vi "tcp 쓰기2.vi"() -> ()   [LabVIEW 2014]
panel:
  out "A":i16[](array[numeric])
  out "에러 출력":errorcluster
  out "문자 2":i16=-19239
  out "문자열":i16[](array[numeric])
  in  "불리언":bool
  out "참 거짓":string
  out "숫자":u32
  in  "stop":bool
  out "문자열":string
  out "Dato Leido":bool[](array[boolean])
  in  "stop 2":bool
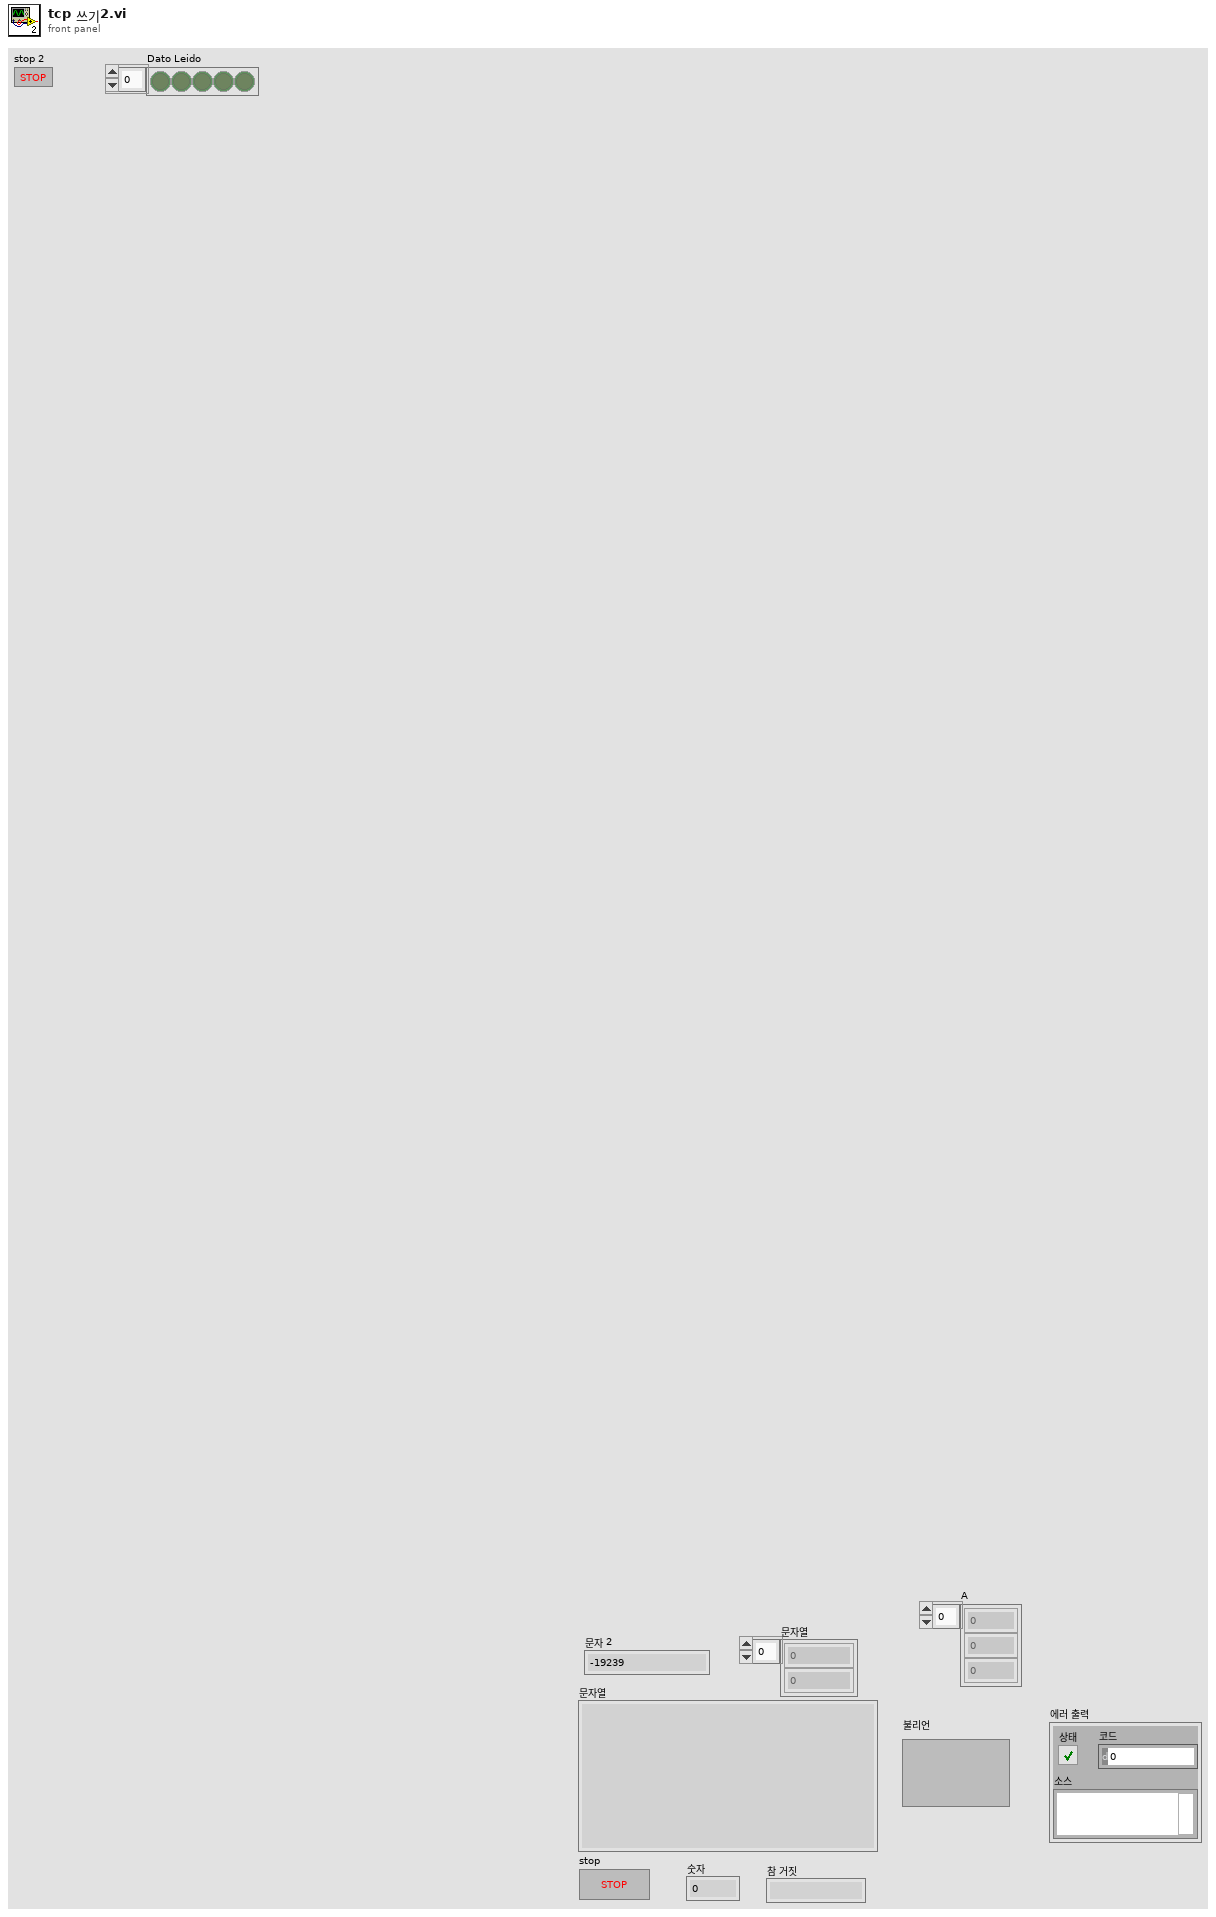
[diagram p1: front panel]
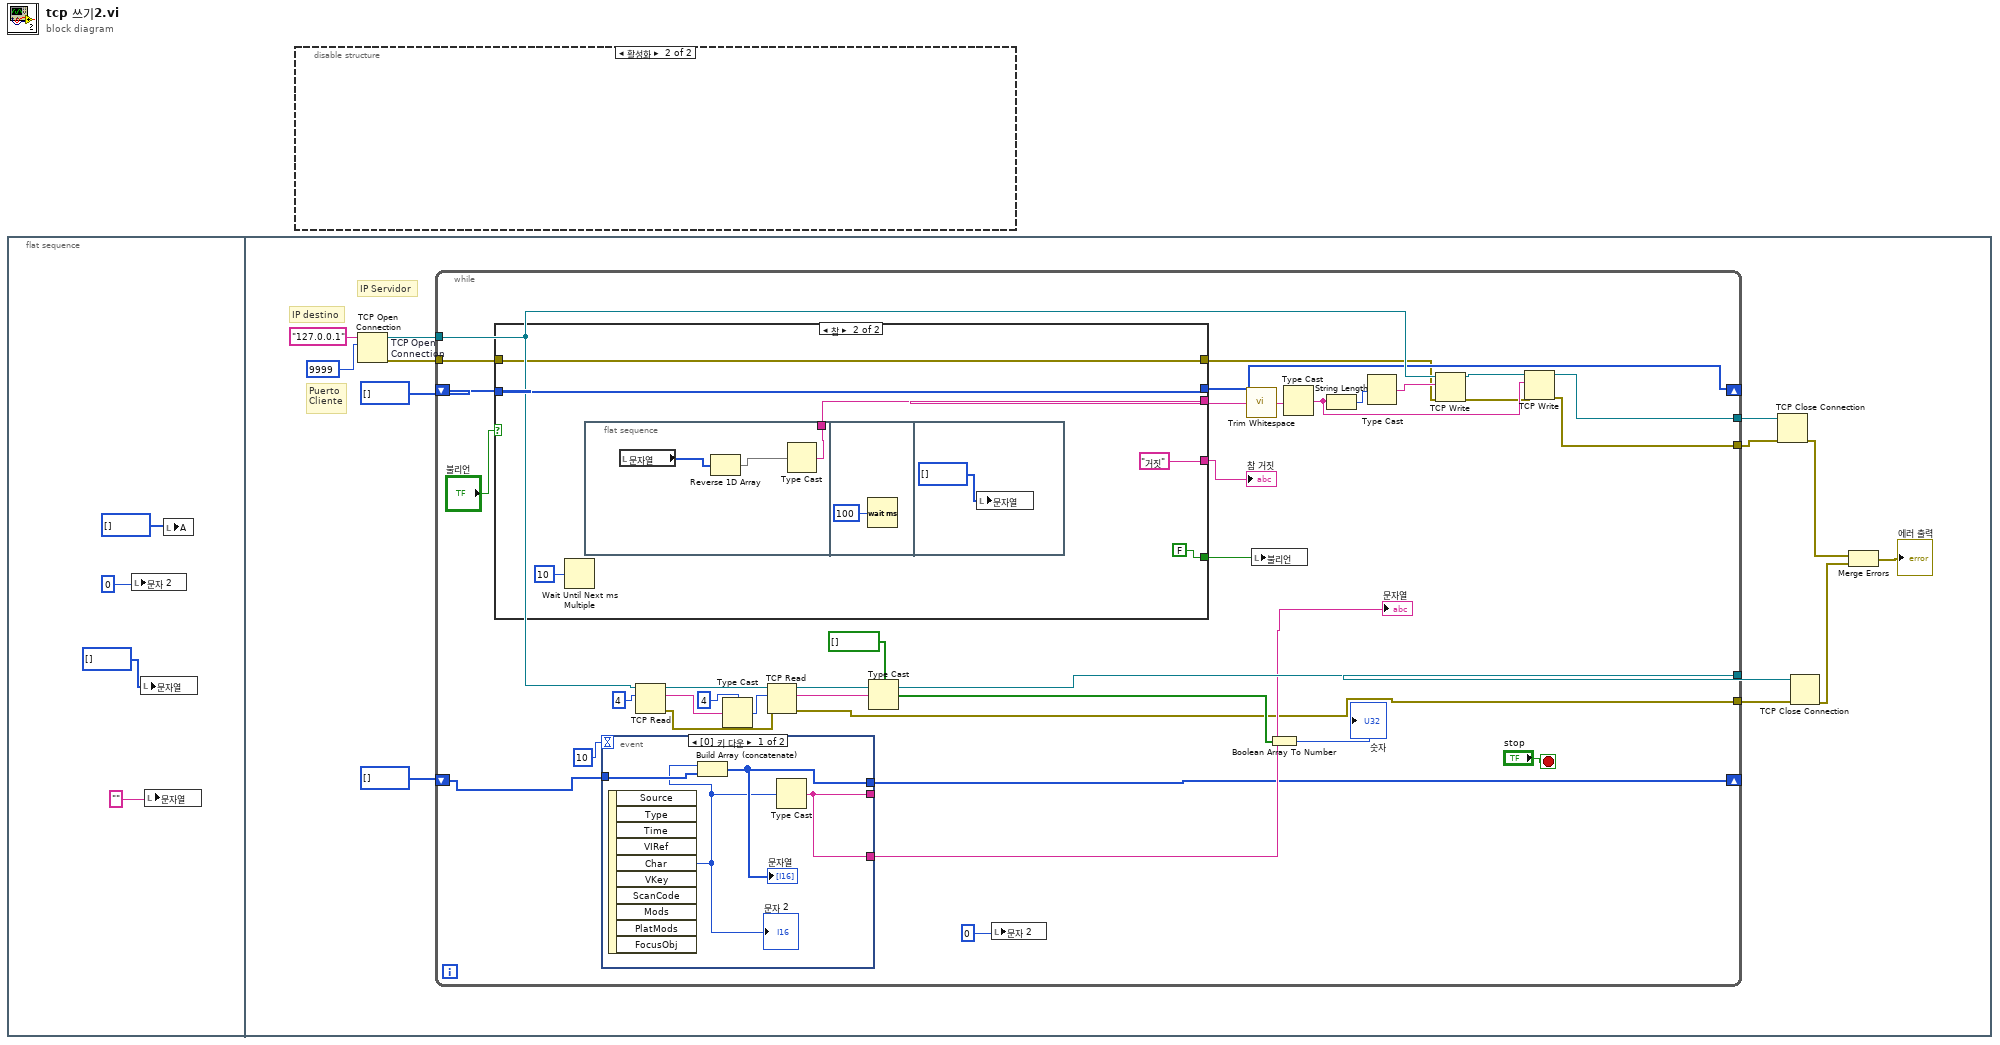
[diagram p0: block diagram]
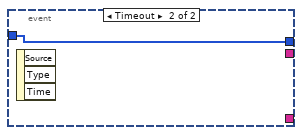
[diagram p2: hidden frame]
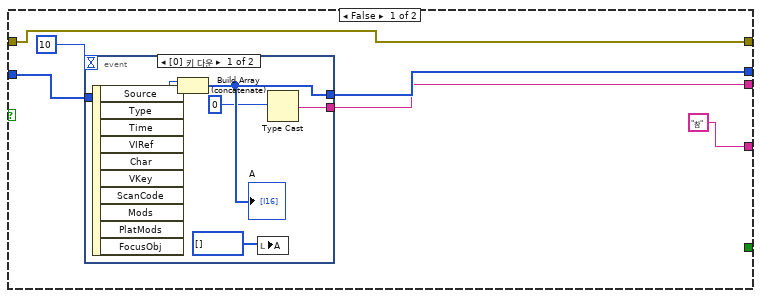
[diagram p3: hidden frame]
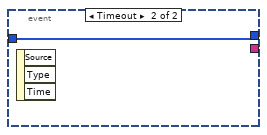
[diagram p4: hidden frame]
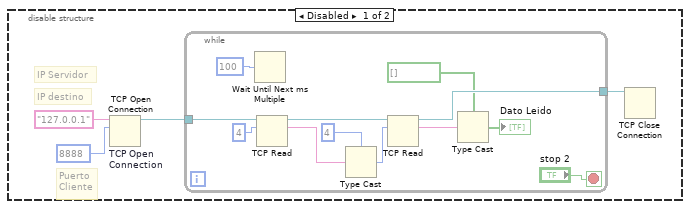
[diagram p5: hidden frame]
diagram:
  n1 = flat-sequence {
    frame #0 {
      n2 = local write "문자 2"(0) -> ()
      n3 = local write "문자열"(i16[] []) -> ()
      n4 = local write "문자열"("") -> ()
      n5 = local write "A"(i16[] []) -> ()
    }
    frame #1 {
      # "Puerto\nCliente"
      # "IP Servidor"
      # "IP destino"
      n6 = TCP Open Connection "TCP Open \nConnection"(address="127.0.0.1", remote port or service name=u16 9999) -> (connection ID=w17:refnum<k5>, error out=w10:errorcluster)  [unwired: 3 in]
      n7 = while {
        tunnel: w17 -> [w44]
        tunnel: [w52] -> w14
        shift-right: [w28] -> _
        shift-left: i16[] [] -> [w51]
        tunnel: [w41] -> w13
        shift-right: [w29] -> _
        shift-left: i16[] [] -> [w30]
        tunnel: w10 -> [w27]
        tunnel: [w24] -> w5
        tunnel: [w22] -> w8
        stop <- "stop" stop-if-true
        n8 = case shown="참" "불리언" {
          tunnel: w51 -> [w63 w76]
          tunnel: [w62 w76] -> w28
          tunnel: [_ FALSE ("불리언")] -> w33
          tunnel: [w60 w72] -> w20
          tunnel: w27 -> [w59 w73]
          tunnel: [w59 w73] -> w26
          tunnel: ["참" "거짓"] -> w18
          frame False {
            n9 = event shown="[0] 키 다운" {
              selector: _ -> [_ _]
              dyn-events: _ -> [_ _]
              timeout: 10 -> [_ _]
              tunnel: [w68 w70] -> w62
              tunnel: w63 -> [w69 w70]
              tunnel: [w66 _] -> w60
              event Key Down {
                n10 = event-data() -> ("Char"=w67:i16)  [unwired: 1 in, 9 out]
                n11 = Build Array (concatenate)(w67, w69) -> (w68:i16[])
                "A" <- w68
                n12 = local write "A"(i16[] []) -> ()
                n13 = Type Cast(x=0) -> (*(type *) &x=w66:string)  [unwired: 1 in]
              }
              event Timeout {
                n14 = event-data() -> ()  [unwired: 1 in, 3 out]
              }
            }
          }
          frame True {
            n15 = Wait Until Next ms Multiple(millisecond multiple=u32 10) -> ()  [unwired: 1 out]
            n16 = flat-sequence {
              tunnel: [w77] -> w72
              frame #0 {
                n17 = local read "문자열"() -> (w78:i16[])
                n18 = Reverse 1D Array(array=w78) -> (reversed array=w79:i16[])
                n19 = Type Cast(x=w79) -> (*(type *) &x=w77:string)  [unwired: 1 in]
              }
              frame #1 {
                n20 = Wait (ms)(milliseconds to wait=u32 100 ("대기 시간(ms)")) -> ()  [unwired: 1 out]
              }
              frame #2 {
                n21 = local write "문자열"(i16[] []) -> ()
              }
            }
          }
        }
        "참 거짓" <- w18
        n22 = event shown="[0] 키 다운" {
          selector: _ -> [_ _]
          dyn-events: _ -> [_ _]
          timeout: 10 -> [_ _]
          tunnel: [w54 w57] -> w29
          tunnel: [w56 _] -> w31
          tunnel: [w56 _] -> _
          tunnel: w30 -> [w55 w57]
          event Key Down {
            n23 = event-data() -> ("Char"=w53:i16)  [unwired: 1 in, 9 out]
            "문자 2" <- w53
            n24 = Build Array (concatenate)(w53, w55) -> (w54:i16[])
            "문자열" <- w54
            n25 = Type Cast(x=w53) -> (*(type *) &x=w56:string)  [unwired: 1 in]
          }
          event Timeout {
            n26 = event-data() -> ()  [unwired: 1 in, 3 out]
          }
        }
        "문자열" <- w31
        n27 = TCP Read(connection ID=w44, bytes to read=4) -> (connection ID out=w49:refnum<k5>, data out=w47:string, error out=w23:errorcluster)  [unwired: 3 in]
        n28 = Type Cast(type=4 ("bytes to read"), x=w47) -> (*(type *) &x=w46:i32)
        n29 = TCP Read(connection ID=w49, bytes to read=w46, error in (no error)=w23) -> (connection ID out=w41:refnum<k5>, data out=w45:string, error out=w22:errorcluster)  [unwired: 2 in]
        n30 = Type Cast(type=bool[] [] ("Dato array"), x=w45) -> (*(type *) &x=w43:bool[])
        n31 = local write "문자 2"(0) -> ()
        n32 = call <vilib>:"Trim Whitespace.vi"("string"=w20) -> ("trimmed string"=w21:string)  [unwired: 1 in]
        n33 = local write "불리언"(w33) -> ()
        n34 = Boolean Array To Number(Boolean array=w43) -> (number=→"숫자":u32)
        n35 = Type Cast(x=w21) -> (*(type *) &x=w35:string)  [unwired: 1 in]
        n36 = String Length(string=w35) -> (length=w36:i32)
        n37 = Type Cast(x=w36) -> (*(type *) &x=w37:string)  [unwired: 1 in]
        n38 = TCP Write(connection ID=w44, data in=w37, error in (no error)=w26) -> (connection ID out=w38:refnum<k5>, error out=w25:errorcluster)  [unwired: 1 in, 1 out]
        n39 = TCP Write(connection ID=w38, data in=w35, error in (no error)=w25) -> (connection ID out=w52:refnum<k5>, error out=w24:errorcluster)  [unwired: 1 in, 1 out]
      }
      n40 = TCP Close Connection(connection ID=w14, error in (no error)=w5) -> (error out=w9:errorcluster)  [unwired: 1 in, 1 out]
      n41 = TCP Close Connection(connection ID=w13, error in (no error)=w8) -> (error out=w6:errorcluster)  [unwired: 1 in, 1 out]
      n42 = Merge Errors(w9, w6) -> (→"에러 출력":errorcluster)
    }
  }
  n43 = disable-structure shown="활성화" {
    frame Disabled {
      # "Puerto\nCliente"
      # "IP Servidor"
      # "IP destino"
      n44 = TCP Open Connection "TCP Open \nConnection"(address="127.0.0.1", remote port or service name=u16 8888) -> (connection ID=w82:refnum<k5>)  [unwired: 3 in, 1 out]
      n45 = while {
        tunnel: w82 -> [w97]
        tunnel: [w95] -> w83
        stop <- "stop 2" stop-if-true
        n46 = Wait Until Next ms Multiple(millisecond multiple=u32 100) -> ()  [unwired: 1 out]
        n47 = TCP Read(connection ID=w97, bytes to read=4) -> (connection ID out=w96:refnum<k5>, data out=w92:string)  [unwired: 3 in, 1 out]
        n48 = Type Cast(type=4 ("bytes to read"), x=w92) -> (*(type *) &x=w91:i32)
        n49 = TCP Read(connection ID=w96, bytes to read=w91) -> (connection ID out=w95:refnum<k5>, data out=w90:string)  [unwired: 3 in, 1 out]
        n50 = Type Cast(type=bool[] [] ("Dato array"), x=w90) -> (*(type *) &x=→"Dato Leido":bool[])
      }
      n51 = TCP Close Connection(connection ID=w83) -> ()  [unwired: 2 in, 2 out]
    }
    frame Enabled {
    }
  }
